vi "UE9 8-Counter Example.vi"() -> ()   [LabVIEW 2021]
panel:
  in  "Case Constant\n(See Context Help)":bool=TRUE
  in  "Reset Counters":bool
  in  "Iteration Inverval (milliseconds)":u32=100
  in  "# of firmware counters to enable":u32=2
  out "Counter1":u32
  out "Counter0":u32
  out "Timer Value Reads":u32[](array[numeric])
  out "Iteration":i32
  in  "error in":errorcluster
  in  "ConnectionType":u16(ring) items=["LJ_ctUSB", "LJ_ctETHERNET"]
  in  "Address":string="1"
  in  "FirstFound":bool=TRUE
  in  "stop":bool
  out "error out":errorcluster
  out "Error Message":string
  # "Enables 0-6 firmware counters (timers) and both hardware counters, then reads\nall at the specified interval.  Timers will be assigned to pins starting with FIO0,\nand the hardware counters will get the next two pins after all timers."
  # "Firmware Counter 0"
  # "Firmware Counter 1"
  # "Firmware Counter 2"
  # "Firmware Counter 3"
  # "Firmware Counter 4"
  # "Firmware Counter 5"
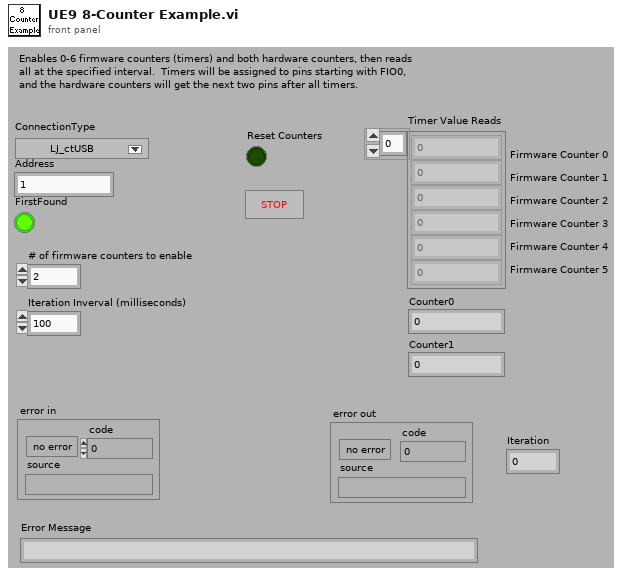
[diagram p1: front panel]
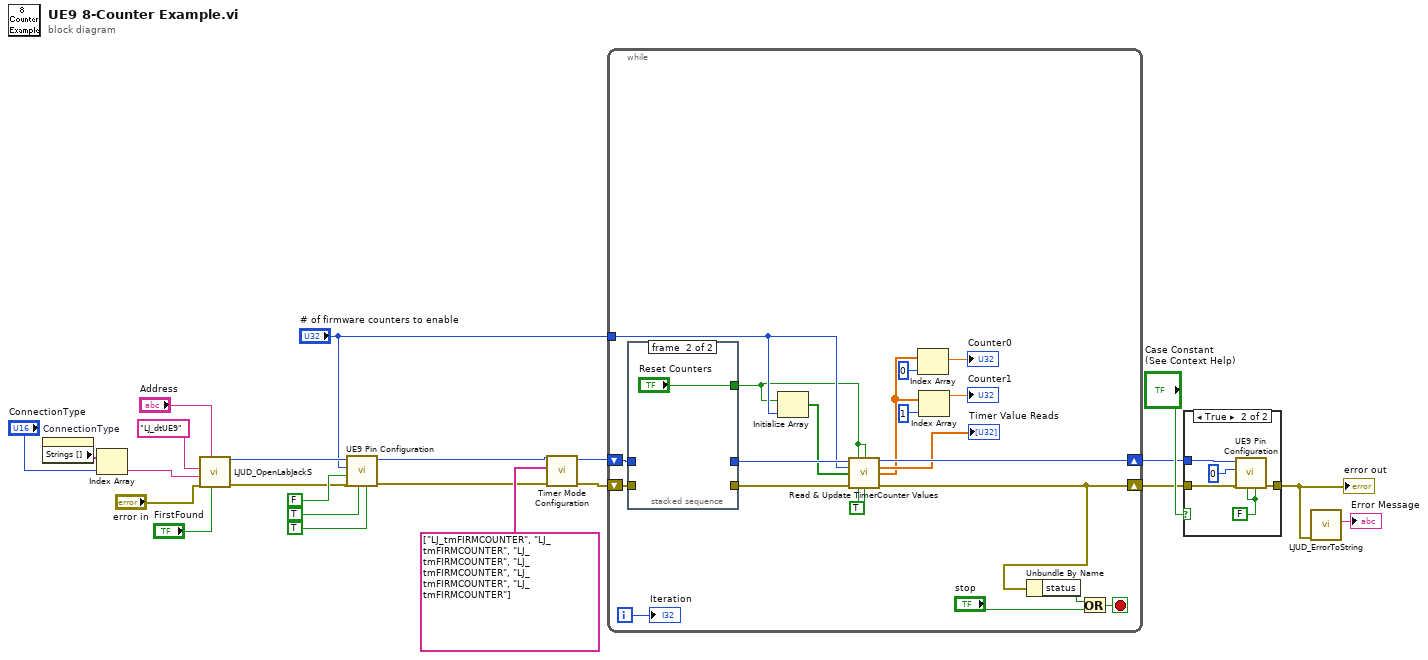
[diagram p0: block diagram]
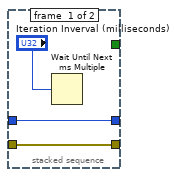
[diagram p3: hidden frame]
diagram:
  n1 = property on="ConnectionType" class="Ring (strict)"() -> ("Strings []"=w14:string[])  [unwired: 2 in, 2 out]
  n2 = Index Array(array=w14, index="ConnectionType") -> (element=w12:string)
  n3 = call "LJUD_OpenLabJackS.vi"("FirstFound"="FirstFound", "Address"="Address", "error in"="error in", "ConnectionType"=w12, "DeviceType"="LJ_dtUE9") -> ("error out"=w6:errorcluster, "Handle"=w7:i32)  [unwired: 4 in, 1 out]
  n4 = call "UE9 Pin Configuration.vi"("Enable Counter1"=TRUE ("Enable Counter0"), "Enable Counter0"=TRUE, "error in"=w6, "Enable DACs"=FALSE ("Enable Counter0"), "Number of Timers Enabled"="# of firmware counters to enable", "Handle In"=w7) -> ("error out"=w4:errorcluster, "Handle Out"=w5:i32)  [unwired: 4 in]
  n5 = call "Timer Mode Configuration.vi"("error in"=w4, "TimerModes"=string[] ["LJ_tmFIRMCOUNTER", "LJ_tmFIRMCOUNTER", "LJ_tmFIRMCOUNTER", "LJ_tmFIRMCOUNTER", "LJ_tmFIRMCOUNTER", "LJ_tmFIRMCOUNTER"], "Handle In"=w5) -> ("error out"=w3:errorcluster, "Handle Out"=w2:i32)  [unwired: 7 in]
  n6 = while {
    shift-right: [w35] -> w19
    shift-left: w2 -> [w43]
    shift-right: [w34] -> w20
    shift-left: w3 -> [w42]
    tunnel: "# of firmware counters to enable" -> [w33]
    i -> [w36]
    stop <- w39 stop-if-true
    w24 = TRUE ("Reset Counter0")
    n7 = stacked-sequence {
      tunnel: [w46 _] -> w41
      tunnel: [w45 _] -> w40
      tunnel: w43 -> [w46 _]
      tunnel: w42 -> [w45 _]
      tunnel: [_ "Reset Counters"] -> w28
      frame #0 {
        n8 = Wait Until Next ms Multiple(millisecond multiple="Iteration Inverval (milliseconds)") -> ()  [unwired: 1 out]
      }
      frame #1 {
      }
    }
    n9 = Initialize Array(w28, w33) -> (w32:bool[])
    n10 = call "Read & Update TimerCounter Values.vi"("Handle In"=w41, "Reset Counter0"=w28, "Reset Counter1"=w28, "# Timers to Read"=w33, "UpdateReset Timers"=w32, "error in"=w40, "Read Counter0"=w24, "Read Counter1"=w24) -> ("Handle Out"=w35:i32, "Timer Value Reads"=→"Timer Value Reads":dbl[], "Counter Value Reads"=w26:dbl[], "error out"=w34:errorcluster)  [unwired: 4 in]
    n11 = Index Array(array=w26, index=0 ("Index")) -> (element=→"Counter0":dbl)
    n12 = Index Array(array=w26, index=1 ("Index")) -> (element=→"Counter1":dbl)
    n13 = Unbundle By Name(w34) -> ("status"=w38:bool)
    n14 = Or(x=w38, y="stop") -> (x .or. y?=w39:bool)
    "Iteration" <- w36
  }
  n15 = case shown="True" "Case Constant\n(See Context Help)" {
    tunnel: w20 -> [w48 w53]
    tunnel: w19 -> [_ w52]
    tunnel: [w48 w50] -> w22
    frame False {
    }
    frame True {
      w49 = FALSE ("Enable Counter0")
      n16 = call "UE9 Pin Configuration.vi"("Enable Counter1"=w49, "Enable Counter0"=w49, "error in"=w53, "Number of Timers Enabled"=u8 0 ("# Timers Enabled"), "Handle In"=w52) -> ("error out"=w50:errorcluster)  [unwired: 5 in, 1 out]
    }
  }
  "error out" <- w22
  n17 = call "LJUD_ErrorToString.vi"("error in"=w22) -> ("String"=→"Error Message":string)  [unwired: 10 in]
